vi "DiffDriveSetSpeedTarget.vi"(9 "Right Speed Ft/Sec":dbl, 10 "Left Speed Ft/Sec":dbl) -> ()   [LabVIEW 2025]
uses:
  DiffDriveGlobals.vi
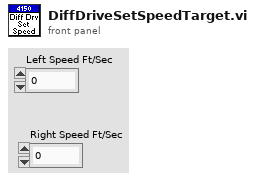
[diagram p1: front panel]
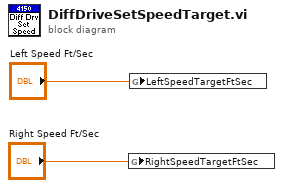
[diagram p0: block diagram]
diagram:
  n1 = global write "DiffDriveGlobals.vi" "RightSpeedTargetFtSec"("Right Speed Ft/Sec") -> ()
  n2 = global write "DiffDriveGlobals.vi" "LeftSpeedTargetFtSec"("Left Speed Ft/Sec") -> ()
